vi "S8300E_BP_4LEDS.vi"() -> ()   [LabVIEW 2011]
panel:
  out "Debug View":string
  out "Turn off CMD-LIST":cluster{string, string, string, string}[](array[cluster])
  out "log msg":string
  out "VISA resource name out":refnum<visa-resource-name>
  out "Turn on CMD-LIST":cluster{string, string, string, string}[](array[cluster])
  out "BEGIN TIME":u32
  out "進行狀況":string
  # "2014-11-14"
  # "Error Code:BP-LED"
  # "S8300E Back Plane 4 LEDs (接UART COM9)"
  # "目檢4 LEDS"
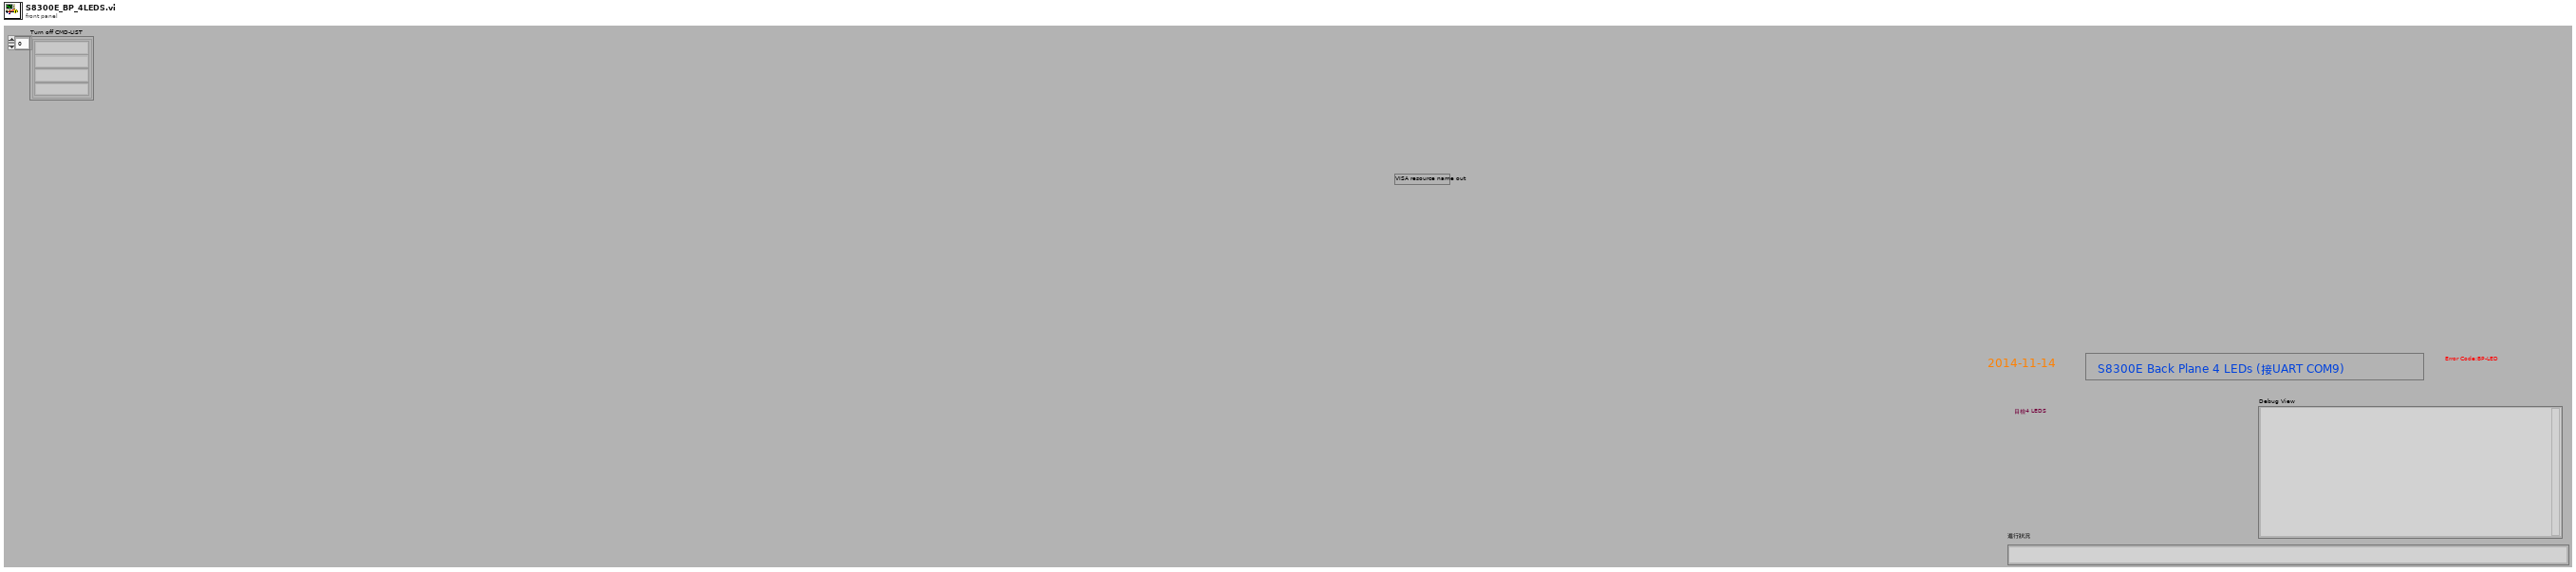
[diagram p1: front panel]
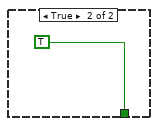
[diagram p6: hidden frame]
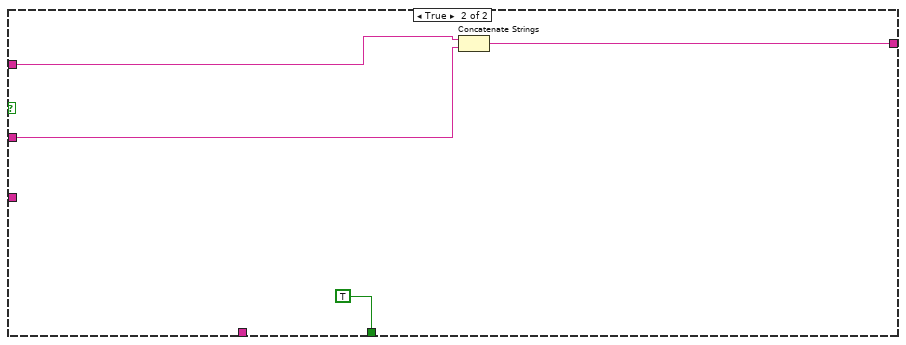
[diagram p8: hidden frame]
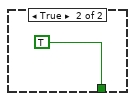
[diagram p11: hidden frame]
diagram:
  n1 = flat-sequence {
    frame #0 {
      n2 = Tick Count (ms)() -> (millisecond timer value=→"BEGIN TIME":u32)
    }
    frame #1 {
      n3 = property on="進行狀況" class="Str"("Blinking"=TRUE) -> ()  [unwired: 2 in, 2 out]
      "進行狀況" <- "進入測試準備中...." ("進行狀況")
      "Debug View" <- ""
    }
    frame #2 {
      n4 = call "SUB_SearchFile_inFolder.vi"("Search Filename in Folder"="S8300E_sfcs_misc.txt") -> ("File Existing True/Flase"=w5:bool)  [unwired: 1 in]
      n5 = case shown="False" w5 {
        frame False {
          n6 = flat-sequence {
            frame #0 {
              n7 = call "Display Message to User"() -> ()  [unwired: 10 in, 2 out]
            }
            frame #1 {
              n8 = call "SUB_Writelog.vi"("Pass/Fail"="Fail:S8300E_BP_4LEDS") -> ()  [unwired: 2 in]
            }
            frame #2 {
              n9 = Quit LabVIEW(quit? (T)=TRUE) -> ()
            }
          }
        }
        frame True {
        }
      }
    }
    frame #3 {
      n10 = Concatenate Strings("./led.sh -w 1 1", "\r") -> (w31:string)
      n11 = Concatenate Strings("./led.sh -w 2 1", "\r") -> (w29:string)
      n12 = Concatenate Strings("./led.sh -w 3 1", "\r") -> (w27:string)
      n13 = Concatenate Strings("./led.sh -w 4 1", "\r") -> (w16:string)
      n14 = Bundle(w29, "PASSED=", "Turn on APP LED .....", "BP-LED") -> (w21:cluster{string, string, string, string})  [unwired: 1 in]
      n15 = Bundle(w27, "PASSED=", "Turn on ACT LED .....", "BP-LED") -> (w20:cluster{string, string, string, string})  [unwired: 1 in]
      n16 = Bundle(w16, "PASSED=", "Turn on OK LED .....", "BP-LED") -> (w9:cluster{string, string, string, string})  [unwired: 1 in]
      n17 = Bundle(w31, "PASSED=", "Turn on ALM LED  .....", "BP-LED") -> (w25:cluster{string, string, string, string})  [unwired: 1 in]
      n18 = Build Array(w25, w21, w20, w9) -> (→"Turn on CMD-LIST":cluster{string, string, string, string}[])
    }
    frame #4 {
      n19 = Concatenate Strings("./led.sh -w 1 0", "\r") -> (w60:string)
      n20 = Concatenate Strings("./led.sh -w 2 0", "\r") -> (w58:string)
      n21 = Concatenate Strings("./led.sh -w 3 0", "\r") -> (w56:string)
      n22 = Concatenate Strings("./led.sh -w 4 0", "\r") -> (w45:string)
      n23 = Bundle(w58, "PASSED=", "Turn off  APP LED .....", "BP-LED") -> (w50:cluster{string, string, string, string})  [unwired: 1 in]
      n24 = Bundle(w56, "PASSED=", "Turn off ACT LED .....", "BP-LED") -> (w49:cluster{string, string, string, string})  [unwired: 1 in]
      n25 = Bundle(w45, "PASSED=", "Turn off  OK LED .....", "BP-LED") -> (w38:cluster{string, string, string, string})  [unwired: 1 in]
      n26 = Bundle(w60, "PASSED=", "Turn off  ALM LED  .....", "BP-LED") -> (w54:cluster{string, string, string, string})  [unwired: 1 in]
      n27 = Build Array(w54, w50, w49, w38) -> (→"Turn off CMD-LIST":cluster{string, string, string, string}[])
    }
    frame #5 {
      n28 = call "SUB_COM1_CLOSE.vi"("VISA resource name"=refnum<visa-resource-name> "COM9") -> ()  [unwired: 3 in]
    }
    frame #6 {
      n29 = case shown="True" TRUE {
        frame False {
        }
        frame True {
          n30 = call "SUB_COM9_INIT.vi"("baud rate"=u32 115200) -> ("VISA resource name out"=w72:refnum<visa-resource-name>)  [unwired: 1 in, 1 out]
          "VISA resource name out" <- w72
          n31 = call "SUB_COM1Wrt.vi"("VISA resource name"=w72, "write buffer"="\r") -> ("duplicate VISA resource name"=w69:refnum<visa-resource-name>)  [unwired: 1 in, 1 out]
          n32 = call "SUB_ContinueCom1Read.vi"("Numeric"=1200, "duplicate VISA resource name 2"=w69) -> ()  [unwired: 1 in, 3 out]
        }
      }
    }
    frame #7 {
      n33 = case shown="True" TRUE {
        frame False {
        }
        frame True {
          n34 = while {
            stop <- w82 stop-if-true
            n35 = local read "VISA resource name out"() -> (w76:refnum<visa-resource-name>)
            n36 = call "SUB_COM1Wrt.vi"("VISA resource name"=w76, "write buffer"="\r") -> ("duplicate VISA resource name"=w81:refnum<visa-resource-name>)  [unwired: 1 in, 1 out]
            n37 = Tick Count (ms)() -> (millisecond timer value=w80:u32)
            n38 = call "SUB_READ_COM1_FindString_timeout.vi"("Find this String"="s8300e_func_test", "Timeout Seccond"=5.0, "Begin time"=w80, "duplicate VISA resource name 2"=w81) -> ("Output String"=w75:string, "Found String"=w77:bool)  [unwired: 1 in, 1 out]
            n39 = local write "Debug View"(w75) -> ()
            n40 = case shown="False" w77 {
              tunnel: [w85 TRUE] -> w82
              tunnel: w75 -> [w84 _]
              frame False {
                n41 = call "SUB_YESNO.vi"("Debug View"=w84, "Status"="UART無正確反應!需有S8300E字串") -> ("yes/no"=w88:enum32{"No Selection", "Yes", "No", "None"})  [unwired: 1 in]
                n42 = Equal?(x=w88, y=enum32{"No Selection", "Yes", "No", "None"}."No") -> (x = y?=w86:bool)
                n43 = case shown="True" w86 {
                  tunnel: [_ w90] -> w85
                  frame False {
                  }
                  frame True {
                    n44 = flat-sequence {
                      tunnel: [w94] -> w90
                      frame #0 {
                        n45 = call "SUB_Writelog.vi"("Pass/Fail"="Fail:S8300E_BP_4LEDS") -> ()  [unwired: 2 in]
                      }
                      frame #1 {
                        n46 = call "SUB_SFCS_SendResult.vi"("ErrorCode"="UART", "PASS_Fail (1/0)"=i8 0) -> ()  [unwired: 1 out]
                      }
                      frame #2 {
                        w94 = TRUE ("quit? (T)")
                        n47 = Quit LabVIEW(quit? (T)=w94) -> ()
                      }
                    }
                  }
                }
              }
              frame True {
              }
            }
          }
        }
      }
    }
    frame #8 {
      n48 = local read "Turn on CMD-LIST"() -> (w99:cluster{string, string, string, string}[])
      n49 = Array Size(array=w99) -> (size(s)=w98:i32)
      n50 = for {
        N: w98 -> [_]
        shift-right: [w101] -> w96
        shift-left: "" -> [w100]
        i -> [w102]
        n51 = while {
          tunnel: w102 -> [w118]
          tunnel: [w105] -> w101
          tunnel: w100 -> [w104]
          stop <- w109 stop-if-true
          n52 = local read "Turn on CMD-LIST"() -> (w117:cluster{string, string, string, string}[])
          n53 = local read "VISA resource name out"() -> (w111:refnum<visa-resource-name>)
          n54 = Index Array(array=w117, index=w118) -> (element=w113:cluster{string, string, string, string})
          n55 = Unbundle(w113) -> (w112:string, w107:string, w108:string, w106:string)
          n56 = call "SUB_COM1Wrt.vi"("VISA resource name"=w111, "write buffer"=w112) -> ("duplicate VISA resource name"=w116:refnum<visa-resource-name>)  [unwired: 1 in, 1 out]
          n57 = Tick Count (ms)() -> (millisecond timer value=w115:u32)
          n58 = call "SUB_READ_COM1_FindString_timeout.vi"("Find this String"=w107, "Timeout Seccond"=2.0, "Begin time"=w115, "duplicate VISA resource name 2"=w116) -> ("Output String"=w103:string, "Found String"=w110:bool)  [unwired: 1 in, 1 out]
          n59 = local write "進行狀況"(w108) -> ()
          n60 = local write "Debug View"(w103) -> ()
          n61 = case shown="False" w110 {
            tunnel: [_ TRUE] -> w109
            tunnel: w108 -> [w125 _]
            tunnel: w103 -> [w124 w135]
            tunnel: w106 -> [w120 _]
            tunnel: [w119 w134] -> w105
            tunnel: w104 -> [w119 w133]
            frame False {
              n62 = Concatenate Strings("與定義不符!" ("string"), w125) -> (w126:string)
              n63 = call "SUB_YESNO.vi"("Debug View"=w124, "Status"=w126) -> ("yes/no"=w123:enum32{"No Selection", "Yes", "No", "None"})  [unwired: 1 in]
              n64 = Equal?(x=w123, y=enum32{"No Selection", "Yes", "No", "None"}."No") -> (x = y?=w121:bool)
              n65 = case shown="True" w121 {
                tunnel: w120 -> [_ w128]
                frame False {
                }
                frame True {
                  n66 = flat-sequence {
                    tunnel: w128 -> [w130]
                    frame #0 {
                      n67 = call "SUB_Writelog.vi"("Pass/Fail"="Fail:S8300E_BP_4LEDS") -> ()  [unwired: 2 in]
                    }
                    frame #1 {
                      n68 = call "SUB_SFCS_SendResult.vi"("ErrorCode"=w130, "PASS_Fail (1/0)"=i8 0) -> ()  [unwired: 1 out]
                    }
                    frame #2 {
                      n69 = Quit LabVIEW(quit? (T)=TRUE) -> ()
                    }
                  }
                }
              }
            }
            frame True {
              n70 = Concatenate Strings(w133, w135) -> (w134:string)
            }
          }
        }
      }
      "log msg" <- w96
    }
    frame #9 {
      (unwired) "4顆LED都有亮?顏色正常?" ("Question:")
      n71 = call "SUB_ASKLEDS_AllOn.vi"() -> ("yes/no"=w137:enum32{"No Selection", "Yes", "No", "None"})  [unwired: 3 in]
      n72 = Equal?(x=w137, y=enum32{"No Selection", "Yes", "No", "None"}."No") -> (x = y?=w138:bool)
      n73 = case shown="True" w138 {
        frame False {
        }
        frame True {
          n74 = flat-sequence {
            frame #0 {
              n75 = call "SUB_Writelog.vi"("Pass/Fail"="Fail:S8300E_BP_4LEDS") -> ()  [unwired: 2 in]
            }
            frame #1 {
              n76 = call "SUB_SFCS_SendResult.vi"("ErrorCode"="BP-LED", "PASS_Fail (1/0)"=i8 0) -> ()  [unwired: 1 out]
            }
            frame #2 {
              n77 = Quit LabVIEW(quit? (T)=TRUE) -> ()
            }
          }
        }
      }
    }
    frame #10 {
      n78 = local read "Turn off CMD-LIST"() -> (w145:cluster{string, string, string, string}[])
      n79 = Array Size(array=w145) -> (size(s)=w144:i32)
      n80 = for {
        N: w144 -> [_]
        i -> [w146]
        n81 = while {
          tunnel: w146 -> [w156]
          stop <- w148 stop-if-true
          n82 = local read "Turn off CMD-LIST"() -> (w155:cluster{string, string, string, string}[])
          n83 = Index Array(array=w155, index=w156) -> (element=w154:cluster{string, string, string, string})
          n84 = local read "VISA resource name out"() -> (w153:refnum<visa-resource-name>)
          n85 = Unbundle(w154) -> (w152:string, w151:string, w150:string)  [unwired: 1 out]
          n86 = call "SUB_COM1Wrt.vi"("VISA resource name"=w153, "write buffer"=w152) -> ("duplicate VISA resource name"=w159:refnum<visa-resource-name>)  [unwired: 1 in, 1 out]
          n87 = Tick Count (ms)() -> (millisecond timer value=w158:u32)
          n88 = local write "進行狀況"(w150) -> ()
          n89 = call "SUB_READ_COM1_FindString_timeout.vi"("Find this String"=w151, "Timeout Seccond"=2.0, "Begin time"=w158, "duplicate VISA resource name 2"=w159) -> ("Output String"=w147:string, "Found String"=w149:bool)  [unwired: 1 in, 1 out]
          n90 = case shown="False" w149 {
            tunnel: [_ TRUE] -> w148
            tunnel: w147 -> [w161 _]
            frame False {
              n91 = call "SUB_YESNO.vi"("Debug View"=w161, "Status"="系統需回PASSED" ("string")) -> ("yes/no"=w164:enum32{"No Selection", "Yes", "No", "None"})  [unwired: 1 in]
              n92 = Equal?(x=w164, y=enum32{"No Selection", "Yes", "No", "None"}."No") -> (x = y?=w162:bool)
              n93 = case shown="True" w162 {
                frame False {
                }
                frame True {
                  n94 = flat-sequence {
                    frame #0 {
                      n95 = call "SUB_Writelog.vi"("Pass/Fail"="Fail:S8300E_BP_4LEDS") -> ()  [unwired: 2 in]
                    }
                    frame #1 {
                      n96 = call "SUB_SFCS_SendResult.vi"("PASS_Fail (1/0)"=i8 0) -> ()  [unwired: 1 in, 1 out]
                    }
                    frame #2 {
                      n97 = Quit LabVIEW(quit? (T)=TRUE) -> ()
                    }
                  }
                }
              }
            }
            frame True {
            }
          }
        }
      }
    }
    frame #11 {
      (unwired) "4顆LED都不亮?" ("Question:")
      n98 = call "SUB_ASKLEDS_AllOff.vi"() -> ("yes/no"=w169:enum32{"No Selection", "Yes", "No", "None"})  [unwired: 3 in]
      n99 = Equal?(x=w169, y=enum32{"No Selection", "Yes", "No", "None"}."No") -> (x = y?=w170:bool)
      n100 = case shown="True" w170 {
        frame False {
        }
        frame True {
          n101 = flat-sequence {
            frame #0 {
              n102 = call "SUB_Writelog.vi"("Pass/Fail"="Fail:S8300E_BP_4LEDS") -> ()  [unwired: 2 in]
            }
            frame #1 {
              n103 = call "SUB_SFCS_SendResult.vi"("ErrorCode"="BP-LED", "PASS_Fail (1/0)"=i8 0) -> ()  [unwired: 1 out]
            }
            frame #2 {
              n104 = Quit LabVIEW(quit? (T)=TRUE) -> ()
            }
          }
        }
      }
    }
    frame #12 {
      n105 = local read "log msg"() -> (w177:string)
      n106 = local read "BEGIN TIME"() -> (w183:u32)
      n107 = Tick Count (ms)() -> (millisecond timer value=w182:u32)
      n108 = call "SUB_CAL_TESTTIME.vi"("Test Item name"="S8300E_BP_4LEDS", "Stop tick time"=w182, "Start tick time"=w183) -> ("Test Time output"=w179:string)  [unwired: 2 in]
      n109 = call "SUB_COM1_CLOSE.vi"("VISA resource name"=refnum<visa-resource-name> "COM9") -> ()  [unwired: 3 in]
      n110 = Concatenate Strings("Pass:S8300E_BP_4LEDS", "\n", w177, w179) -> (w180:string)
      n111 = call "SUB_Writelog.vi"("Pass/Fail"=w180) -> ()  [unwired: 2 in]
    }
    frame #13 {
      n112 = Quit LabVIEW(quit? (T)=TRUE ("stop? (T)")) -> ()
    }
  }
